vi "fpga_Timer.vi"(0 "status in":T2, 1 "timing values in":T3, 5 "pick-up signal? (F)":bool, 7 "time delay settings":T1, 9 "input valid?":bool, 11 "trip signal in":bool, 12 "instantaneous reset after tripping? (F)":bool) -> (3 "timing values out":T3, 4 "status out":T2, 15 "trip signal out":bool)   [LabVIEW 2012, in "NI_EP_Protection_FPGA.lvlib"]
uses:
  <vilib>/addons/Electrical Power/Protection/NI_EP_Protection_FPGA.lvlib
  <vilib>/addons/Electrical Power/Protection/Definite Time Delay/subVIs/fpga_Timer Feedback Var.ctl
  <vilib>/addons/Electrical Power/Protection/Definite Time Delay/subVIs/fpga_State.ctl
  <vilib>/addons/Electrical Power/Protection/Definite Time Delay/subVIs/fpga_Time Delay Cfg.ctl
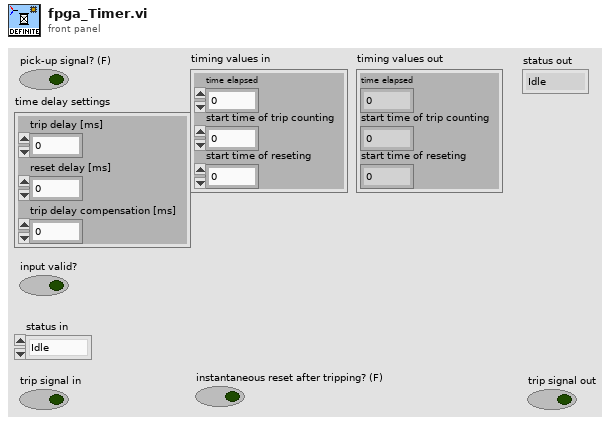
[diagram p1: front panel]
types:
  T1 = typedef "NI_EP_Protection_FPGA.lvlib/fpga_Time Delay Cfg.ctl" = cluster{"trip delay [ms]":u32, "reset delay [ms]":u32, "trip delay compensation [ms]":u32}
  T2 = typedef "NI_EP_Protection_FPGA.lvlib/fpga_State.ctl" = enum16{"Idle", "Trip Counting", "Tripped", "Reset Counting"}
  T3 = typedef "NI_EP_Protection_FPGA.lvlib/fpga_Timer Feedback Var.ctl" = cluster{"time elapsed":u32, "start time of trip counting":u32, "start time of reseting":u32}
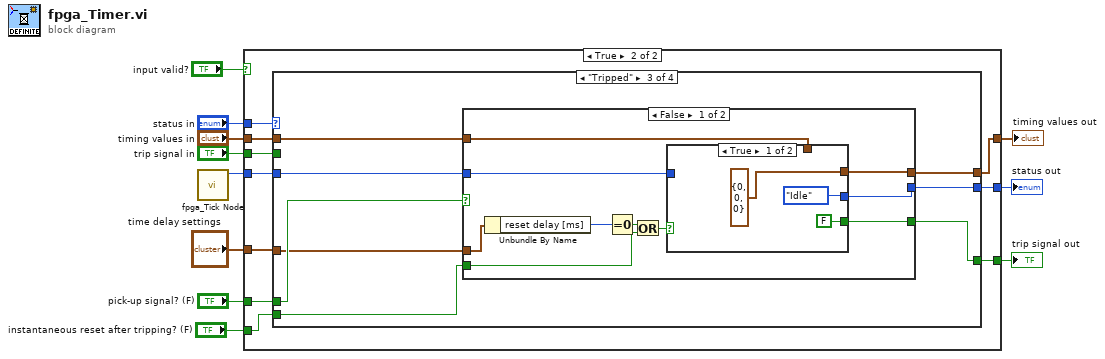
[diagram p0: block diagram]
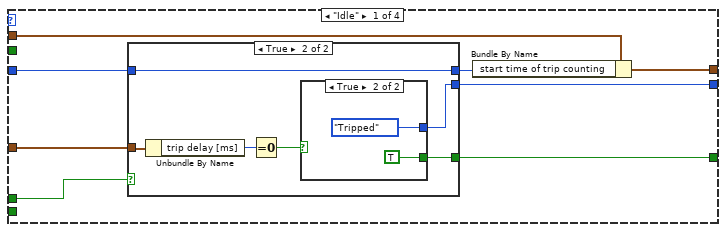
[diagram p3: hidden frame]
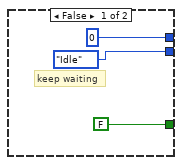
[diagram p4: hidden frame]
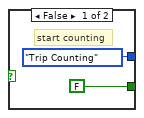
[diagram p5: hidden frame]
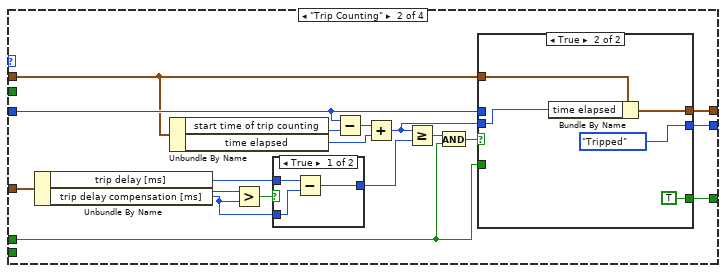
[diagram p6: hidden frame]
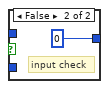
[diagram p7: hidden frame]
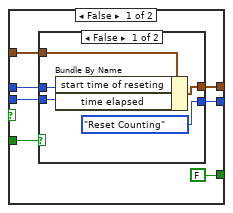
[diagram p8: hidden frame]
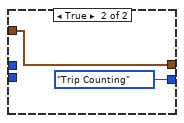
[diagram p9: hidden frame]
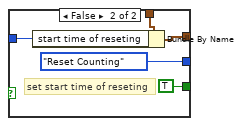
[diagram p10: hidden frame]
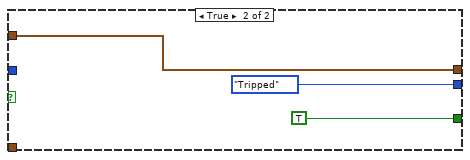
[diagram p11: hidden frame]
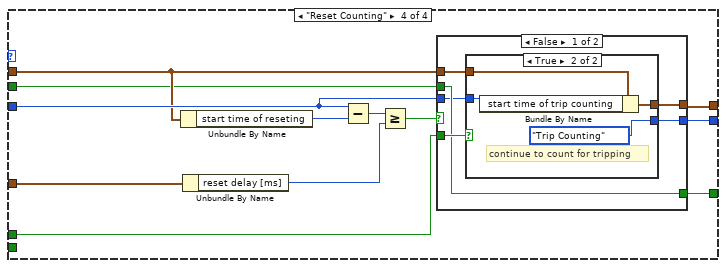
[diagram p12: hidden frame]
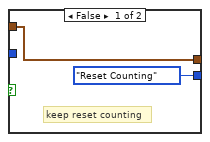
[diagram p13: hidden frame]
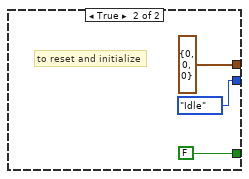
[diagram p14: hidden frame]
diagram:
  n1 = call <vilib>:"fpga_Tick Node.vi"() -> ("millisecond timer value"=w4:u32)  [unwired: 11 in]
  n2 = case shown="True" "input valid?" {
    tunnel: "timing values in" -> [w13 w24]
    tunnel: "status in" -> [w14 w23]
    tunnel: [w13 w22] -> w9
    tunnel: [w14 w21] -> w8
    tunnel: "trip signal in" -> [w12 w20]
    tunnel: [w12 w19] -> w6
    tunnel: "pick-up signal? (F)" -> [_ w18]
    tunnel: w4 -> [_ w17]
    tunnel: "time delay settings" -> [_ w16]
    tunnel: "instantaneous reset after tripping? (F)" -> [_ w15]
    frame False {
    }
    frame True {
      n3 = case shown="\"Tripped\"" w23 {
        tunnel: w18 -> [w32 w55 w93 w117]
        tunnel: [w29 w62 w91 w124] -> w21
        tunnel: [w25 w61 w88 w125] -> w19
        tunnel: w20 -> [_ _ _ w116]
        tunnel: w24 -> [w30 w49 w90 w121]
        tunnel: [w31 w50 w89 w120] -> w22
        tunnel: w17 -> [w28 w54 w92 w122]
        tunnel: w16 -> [w26 w48 w87 w119]
        tunnel: w15 -> [_ _ w86 _]
        frame "Idle" {
          n4 = case shown="True" w32 {
            tunnel: [fpga_State."Idle" w36] -> w29
            tunnel: w28 -> [_ w41]
            tunnel: [u32 0 ("Tick Count(mSec)") w41] -> w27
            tunnel: w26 -> [_ w39]
            tunnel: [FALSE ("trip?") w37] -> w25
            frame False {
              # "keep waiting"
            }
            frame True {
              n5 = Unbundle By Name(w39) -> ("trip delay [ms]"=w40:u32)
              n6 = Equal To 0?(x=w40) -> (x = 0?=w38:bool)
              n7 = case shown="True" w38 {
                tunnel: [FALSE ("trip?") TRUE ("trip?")] -> w37
                tunnel: [fpga_State."Trip Counting" fpga_State."Tripped"] -> w36
                frame False {
                  # "start counting"
                }
                frame True {
                }
              }
            }
          }
          n8 = Bundle By Name(cluster=w30, "start time of trip counting"=w27) -> (w31:T3)
        }
        frame "Trip Counting" {
          n9 = Unbundle By Name(w48) -> ("trip delay [ms]"=w47:u32, "trip delay compensation [ms]"=w46:u32)
          n10 = Unbundle By Name(w49) -> ("start time of trip counting"=w53:u32, "time elapsed"=w52:u32)
          n11 = Greater?(x=w47, y=w46) -> (0:w57:bool)
          n12 = case shown="True" w57 {
            tunnel: w47 -> [w65 _]
            tunnel: w46 -> [w64 _]
            tunnel: [w63 u32 0] -> w51
            frame True {
              n13 = Subtract(x=w65, y=w64) -> (x-y=w63:u32)
            }
            frame False {
              # "input check"
            }
          }
          n14 = Subtract(x=w54, y=w53) -> (x-y=w58:u32)
          n15 = Add(x=w58, y=w52) -> (x+y=w56:u32)
          n16 = Greater Or Equal?(x=w56, y=w51) -> (x >= y?=w59:bool)
          n17 = And(x=w59, y=w55) -> (x .and. y?=w60:bool)
          n18 = case shown="True" w60 {
            tunnel: [w72 fpga_State."Tripped"] -> w62
            tunnel: [FALSE ("trip?") TRUE ("trip?")] -> w61
            tunnel: w55 -> [w73 _]
            tunnel: w56 -> [w71 w81]
            tunnel: w54 -> [w70 _]
            tunnel: [w68 w82] -> w50
            tunnel: w49 -> [w67 w83]
            frame False {
              n19 = case shown="False" w73 {
                tunnel: [fpga_State."Reset Counting" fpga_State."Trip Counting"] -> w72
                tunnel: w71 -> [w76 _]
                tunnel: w70 -> [w77 _]
                tunnel: [w75 w79] -> w68
                tunnel: w67 -> [w74 w79]
                frame False {
                  n20 = Bundle By Name(cluster=w74, "start time of reseting"=w77, "time elapsed"=w76) -> (w75:T3)
                }
                frame True {
                }
              }
            }
            frame True {
              n21 = Bundle By Name(cluster=w83, "time elapsed"=w81) -> (w82:T3)
            }
          }
        }
        frame "Tripped" {
          n22 = case shown="False" w93 {
            tunnel: [w103 fpga_State."Tripped"] -> w91
            tunnel: w92 -> [w100 _]
            tunnel: w90 -> [w101 w113]
            tunnel: [w102 w113] -> w89
            tunnel: [w99 TRUE ("trip?")] -> w88
            tunnel: w87 -> [w97 _]
            tunnel: w86 -> [w95 _]
            frame False {
              n23 = Unbundle By Name(w97) -> ("reset delay [ms]"=w98:u32)
              n24 = Equal To 0?(x=w98) -> (x = 0?=w96:bool)
              n25 = Or(x=w96, y=w95) -> (x .or. y?=w94:bool)
              n26 = case shown="True" w94 {
                tunnel: [fpga_State."Idle" fpga_State."Reset Counting"] -> w103
                tunnel: [T3 {"time elapsed"=0, "start time of trip counting"=0, "start time of reseting"=0} ("timer in") w110] -> w102
                tunnel: w101 -> [_ w109]
                tunnel: w100 -> [_ w108]
                tunnel: [FALSE TRUE] -> w99
                frame True {
                }
                frame False {
                  # "set start time of reseting"
                  n27 = Bundle By Name(cluster=w109, "start time of reseting"=w108) -> (w110:T3)
                }
              }
            }
            frame True {
            }
          }
        }
        frame "Reset Counting" {
          n28 = Unbundle By Name(w121) -> ("start time of reseting"=w123:u32)
          n29 = Unbundle By Name(w119) -> ("reset delay [ms]"=w118:u32)
          n30 = Subtract(x=w122, y=w123) -> (x-y=w126:u32)
          n31 = Greater Or Equal?(x=w126, y=w118) -> (x >= y?=w115:bool)
          n32 = case shown="False" w115 {
            tunnel: [w130 FALSE ("trip?")] -> w125
            tunnel: w116 -> [w130 _]
            tunnel: [w131 fpga_State."Idle"] -> w124
            tunnel: w117 -> [w132 _]
            tunnel: w122 -> [w129 _]
            tunnel: w121 -> [w128 _]
            tunnel: [w127 T3 {"time elapsed"=0, "start time of trip counting"=0, "start time of reseting"=0} ("timer in")] -> w120
            frame False {
              n33 = case shown="True" w132 {
                tunnel: [fpga_State."Reset Counting" fpga_State."Trip Counting"] -> w131
                tunnel: w129 -> [_ w138]
                tunnel: w128 -> [w133 w137]
                tunnel: [w133 w136] -> w127
                frame False {
                  # "keep reset counting"
                }
                frame True {
                  # "continue to count for tripping"
                  n34 = Bundle By Name(cluster=w137, "start time of trip counting"=w138) -> (w136:T3)
                }
              }
            }
            frame True {
              # "to reset and initialize"
            }
          }
        }
      }
    }
  }
  "timing values out" <- w9
  "status out" <- w8
  "trip signal out" <- w6
